vi "Get Events.vi"(11 "Create Test Channel View in":refnum<class "Create Test Channel View.lvclass">) -> (2 "Events":T1, 3 "Create Test Channel View out":refnum<class "Create Test Channel View.lvclass">)   [LabVIEW 2013, in "Create Test Channel View.lvlib" / "Create Test Channel View.lvclass"]
uses:
  Create Test Channel View.lvclass
  Typedef/Events.ctl
  Create Test Channel View.lvclass/Create Test Channel View.ctl
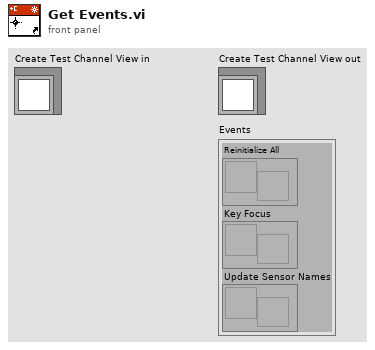
[diagram p1: front panel]
types:
  T1 = typedef "Create Test Channel View.lvlib/Create Test Channel View.lvclass/Events.ctl" = cluster{"Reinitialize All":refnum<user-event>, "Key Focus":refnum<user-event>, "Update Sensor Names":refnum<user-event>}
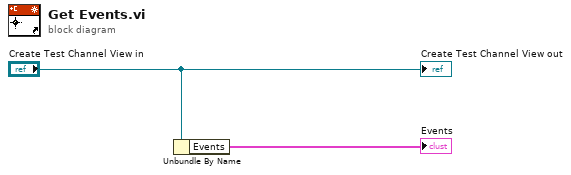
[diagram p0: block diagram]
diagram:
  n1 = Unbundle By Name("Create Test Channel View in") -> ("Events"=→"Events":T1)
  "Create Test Channel View out" <- "Create Test Channel View in"
